vi "Extension to Mode.vi"(11 "lowercase file extension":string) -> (3 "Mode":T1)   [LabVIEW 2019, in "Build.lvlib"]
uses:
  Build.lvlib
  Typedefs/Build Type--enum.ctl
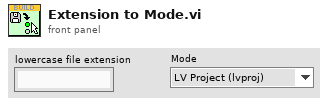
[diagram p1: front panel]
types:
  T1 = typedef "Build.lvlib/Build Type--enum.ctl" = enum16{"LV Project (lvproj)", "Build Spec (vipb)", "Package (vip)"}
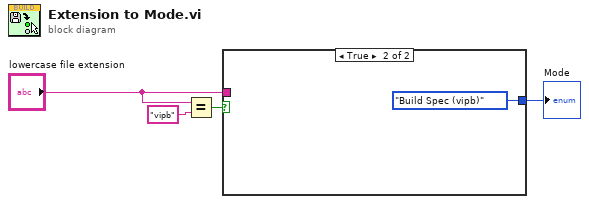
[diagram p0: block diagram]
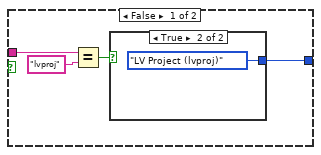
[diagram p2: hidden frame]
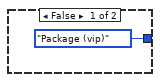
[diagram p3: hidden frame]
diagram:
  n1 = Equal?(x="lowercase file extension", y="vipb") -> (x = y?=w3:bool)
  n2 = case shown="True" w3 {
    tunnel: [w5 Build_Type--enum."Build Spec (vipb)" ("Mode")] -> w4
    tunnel: "lowercase file extension" -> [w7 _]
    frame False {
      n3 = Equal?(x=w7, y="lvproj") -> (x = y?=w6:bool)
      n4 = case shown="True" w6 {
        tunnel: [Build_Type--enum."Package (vip)" ("Mode") Build_Type--enum."LV Project (lvproj)" ("Mode")] -> w5
        frame False {
        }
        frame True {
        }
      }
    }
    frame True {
    }
  }
  "Mode" <- w4
